vi "File_Stop.vi"(8 "error in":errorcluster, 10 "Version":string, 11 "File.lvclass (IN)":refnum<class "File.lvclass">) -> (0 "error out":errorcluster, 3 "File.lvclass (OUT)":refnum<class "File.lvclass">)   [LabVIEW 2013, in "File.lvclass"]
uses:
  File.lvclass
  File.lvclass/File.ctl
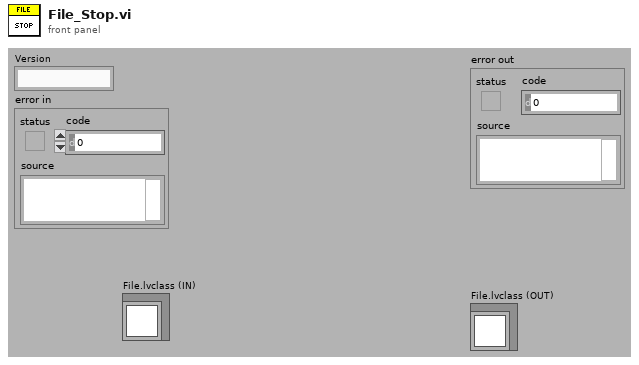
[diagram p1: front panel]
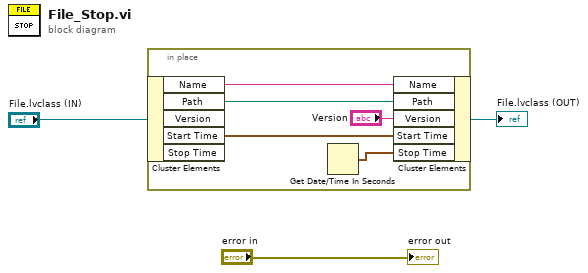
[diagram p0: block diagram]
diagram:
  n1 = in-place {
    n2 = in-place-cluster #1("File.lvclass (IN)") -> ("Name"=w8:string, "Path"=w7:path, "Start Time"=w5:timestamp)  [unwired: 2 out]
    n3 = Get Date/Time In Seconds() -> (seconds since 1Jan1904=w4:timestamp)
    n4 = in-place-cluster #1("Name"=w8, "Path"=w7, "Version"="Version", "Start Time"=w5, "Stop Time"=w4) -> (→"File.lvclass (OUT)":refnum<class "File.lvclass">)
  }
  "error out" <- "error in"
